vi "ZigZagTactic.vi"(6 "IndexInVector":dbl, 8 "error in (no error)":errorcluster, 9 "Game in":refnum<class "Game.lvclass">, 10 "Robot":refnum<class "Robot.lvclass">, 11 "ZigZagTactic in":refnum<class "ZigZagTactic.lvclass">) -> (0 "error out":errorcluster, 2 "Robot out":refnum<class "Robot.lvclass">, 3 "ZigZagTactic out":refnum<class "ZigZagTactic.lvclass">)   [LabVIEW 2018, in "ZigZagTactic.lvclass"]
uses:
  ZigZagTactic.lvclass
  C:/Users/Gustavo/Desktop/RoboIME/SimplePass/SSL_AI/Tactic_class/Tactic.lvclass
  Robot_class/Robot.lvclass
  Game_class/Game.lvclass
  Tactic_class/Tactic.lvclass/Tactic.ctl
  Robot_class/tactics.ctl
  Skillbook_class/Skillbook.lvclass/Skillbook.ctl
  ZigZagTactic.lvclass/ZigZagTactic.ctl
  Robot_class/Robot.lvclass/Robot.ctl
  Skillbook_class/Read ZigZagSkill.vi
  Tactic_class/Read Skillbook.vi
  Robot_class/Write tactic.vi
  Write States.vi
  Skillbook_class/Skillbook.lvclass
  ZigZagSkill_class/ZigZagSkill.lvclass
panel:
  out "x .or. y?":bool
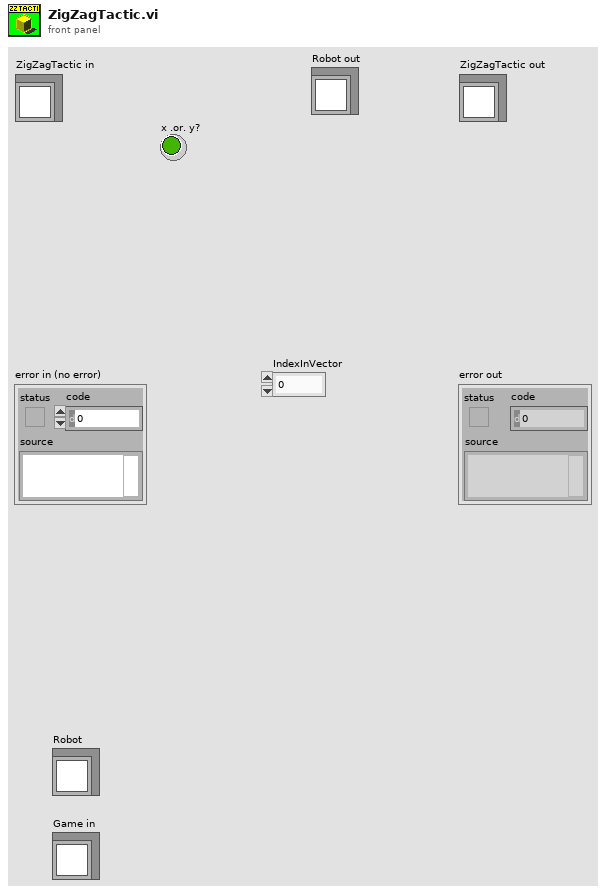
[diagram p1: front panel]
types:
  T1 = typedef "tactics.ctl" = enum16{"PenaltyAttacker", "PassObserver", "PenaltyDefense", "Test", "DefendGoal", "Marker", "FollowAttacker", "DefendArea", "Shoot", "AttackerAimGoal", "AttackerBallOutOfField", "AttackerBlock", "AttackerStop", "Duelist", "Halt", "ZigZag", "GoTo", "Timeout", "KickToPassReceiver", "PositionToReceivePass", "PassReceiver", "WaitPass"}
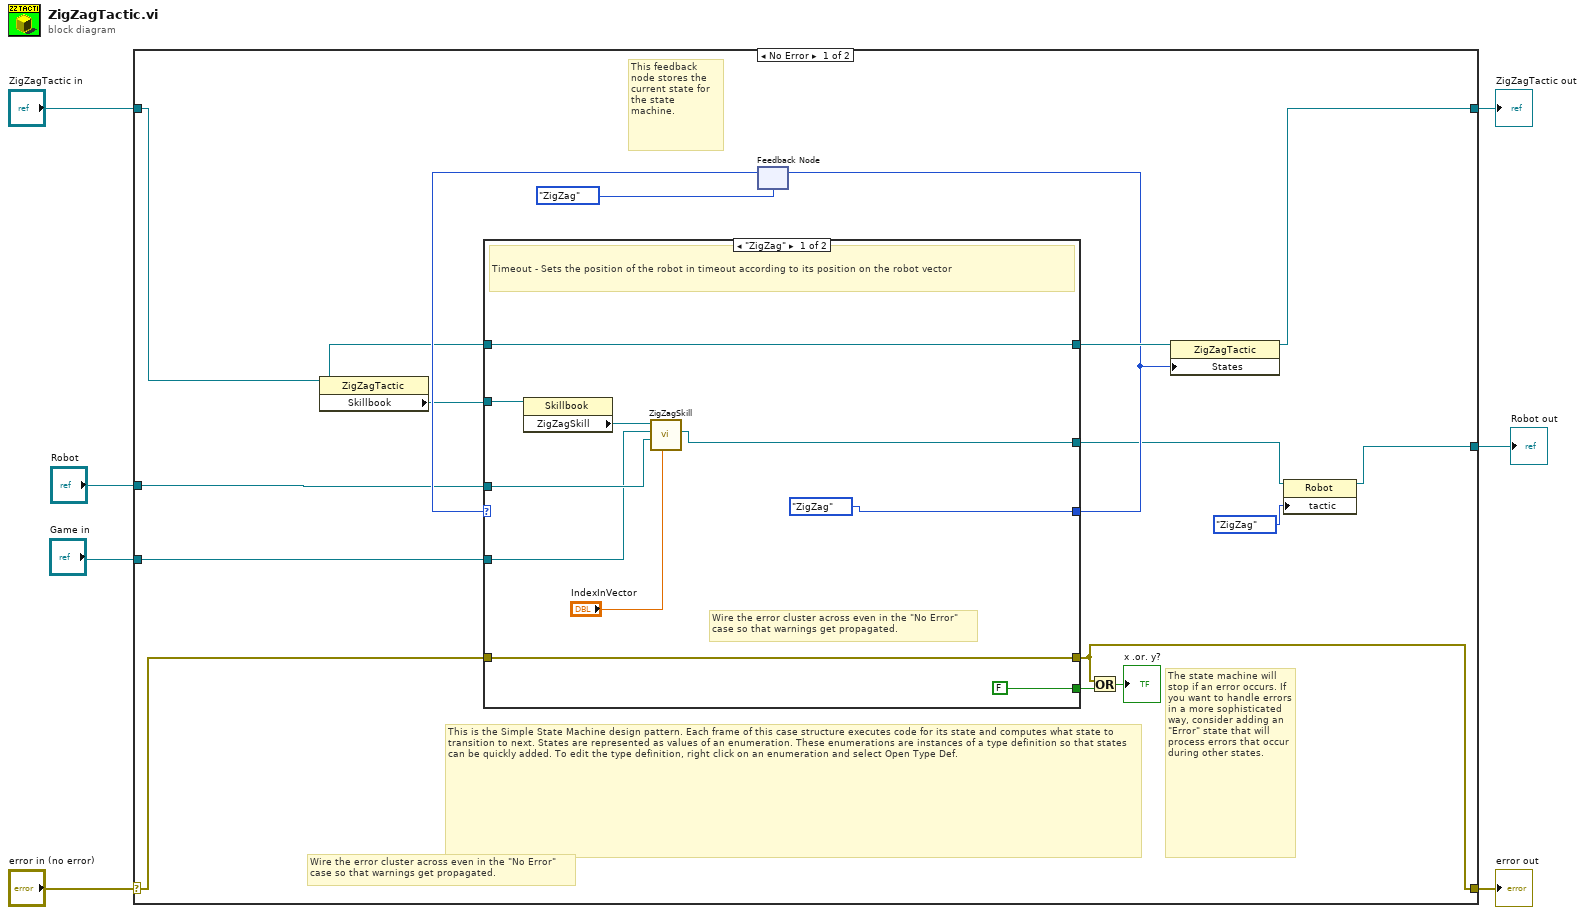
[diagram p0: block diagram]
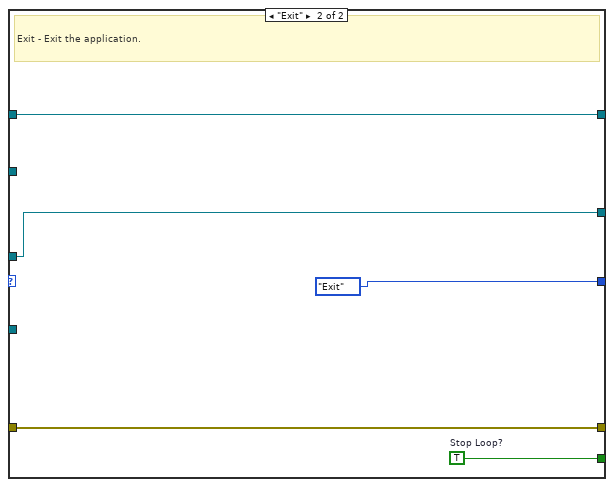
[diagram p2: hidden frame]
diagram:
  n1 = case shown="No Error" "error in (no error)" {
    selector: "error in (no error)" -> [w17 w41]
    tunnel: [w18 w41] -> w6
    tunnel: [w15 w40] -> w4
    tunnel: "ZigZagTactic in" -> [w16 w40]
    tunnel: [w8 w39] -> w3
    tunnel: "Robot" -> [w14 w39]
    tunnel: "Game in" -> [w13 _]
    frame No Error {
      # "The state machine will stop if an error occurs. If you want to handle errors in a more sophisticated way, consider adding an \"Error\" state that will process errors that occur during other states."
      # "This feedback node stores the current state for the state machine."
      # "This is the Simple State Machine design pattern. Each frame of this case structure executes code for its state and computes what state to transition to next. States are represented as values of an enumeration. These enumerations are instances of a type definition so that states can be quickly added. To edit the type definition, right click on an enumeration and select Open Type Def."
      # "Wire the error cluster across even in the \"No Error\"\ncase so that warnings get propagated."
      # "Wire the error cluster across even in the \"No Error\"\ncase so that warnings get propagated."
      n2 = property class="ZigZagTactic"(reference=w16) -> ("Skillbook"=w20:refnum<class "Skillbook.lvclass">)  [unwired: 1 in, 2 out]
      n3 = feedback #1(enum16{"ZigZag", "Exit"}."ZigZag" ("States")) -> (w21:enum16{"ZigZag", "Exit"})
      n4 = case shown="\"ZigZag\"" w21 {
        tunnel: [enum16{"ZigZag", "Exit"}."ZigZag" ("States") enum16{"ZigZag", "Exit"}."Exit" ("States")] -> w11
        tunnel: [FALSE ("Stop Loop?") w38] -> w23
        tunnel: w17 -> [w32 w37]
        tunnel: [w32 w37] -> w18
        tunnel: w20 -> [w31 _]
        tunnel: w14 -> [w28 w36]
        tunnel: [w27 w36] -> w9
        tunnel: [w30 w35] -> w19
        tunnel: w16 -> [w30 w35]
        tunnel: w13 -> [w26 _]
        frame "ZigZag" {
          # "Timeout - Sets the position of the robot in timeout according to its position on the robot vector"
          n5 = property class="Skillbook"(reference=w31) -> ("ZigZagSkill"=w29:refnum<class "ZigZagSkill.lvclass">)  [unwired: 1 in, 2 out]
          n6 = call-dynamic "ZigZagSkill.vi"("ZigZag Number"="IndexInVector", "Robot"=w28, "Game in"=w26, "ZigZagSkill in"=w29) -> ("Robot out"=w27:refnum<class "Robot.lvclass">)  [unwired: 4 in, 3 out]
        }
        frame "Exit" {
          w38 = TRUE  # Stop Loop?
          # "Exit - Exit the application."
        }
      }
      n7 = feedback-in #1(w11) -> ()
      n8 = Or(x=w18, y=w23) -> (x .or. y?=→"x .or. y?":bool)
      n9 = property class="ZigZagTactic"(reference=w19, "States"=w11) -> (reference out=w15:refnum<class "ZigZagTactic.lvclass">)  [unwired: 1 in, 1 out]
      n10 = property class="Robot"(reference=w9, "tactic"=tactics."ZigZag") -> (reference out=w8:refnum<class "Robot.lvclass">)  [unwired: 1 in, 1 out]
    }
    frame Error {
    }
  }
  "error out" <- w6
  "ZigZagTactic out" <- w4
  "Robot out" <- w3
